vi "MS-2000 Stage Engine.vi"(0 "MS-2000 Notifier Name":string="MS2000", 11 "COM Port":string[](array[string])) -> ()   [LabVIEW 2020]
uses:
  Stages Controls/Stage Notifier Element.ctl
  Stages Controls/Stage Actions.ctl
  Stages Controls/Stage Status.ctl
  <vilib>/Instr/_visa.llb/VISA Configure Serial Port (Instr).vi
panel:
  out "Last Error":errorcluster
  in  "Get Position":bool
  in  "XY Step Size (µm)":dbl format="%#_4g"
  in  "Y Position (µm)":dbl format="%#_4g"
  in  "X Position (µm)":dbl format="%#_4g"
  in  "Home":bool
  in  "Right":bool
  in  "Left":bool
  in  "Down":bool
  in  "Halt":bool
  in  "Up":bool
  in  "Quit":bool
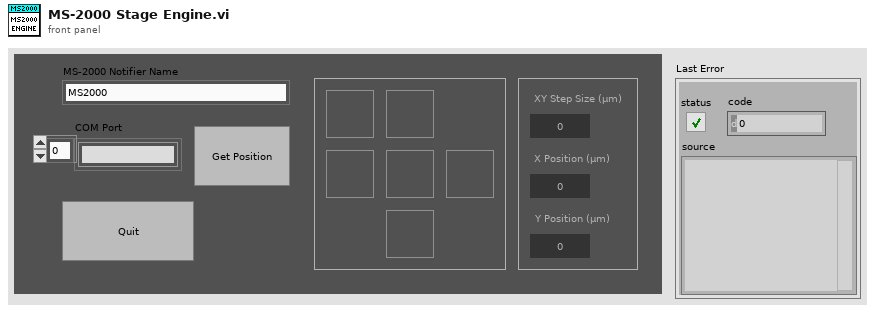
[diagram p1: front panel]
types:
  T1 = typedef "Stage Notifier Element.ctl" = cluster{"Action":T2, "Axis":bool[], "Setpoint":dbl[], "Velocity":dbl, "Cmd Recvd?":bool, "Position":dbl[], "Status":T3, "Misc":variant}
  T2 = typedef "Stage Actions.ctl" = enum16{"Get Position", "MVR", "MOVE", "HALT", "ONTARGET", "ERROR", "REFERENCE", "INIT", "VELOCITY", "STATUS", "EXIT", "HOME", "ZEROPOS", "NANOPOS", "ANALOG", "QUIT"}
  T3 = typedef "Stage Status.ctl" = enum16{"Error", "Abort", "Busy", "On Target"}
  T4 = enum32{"Invalid", "Standard", "Closed", "Hidden", "Minimized", "Maximized"}
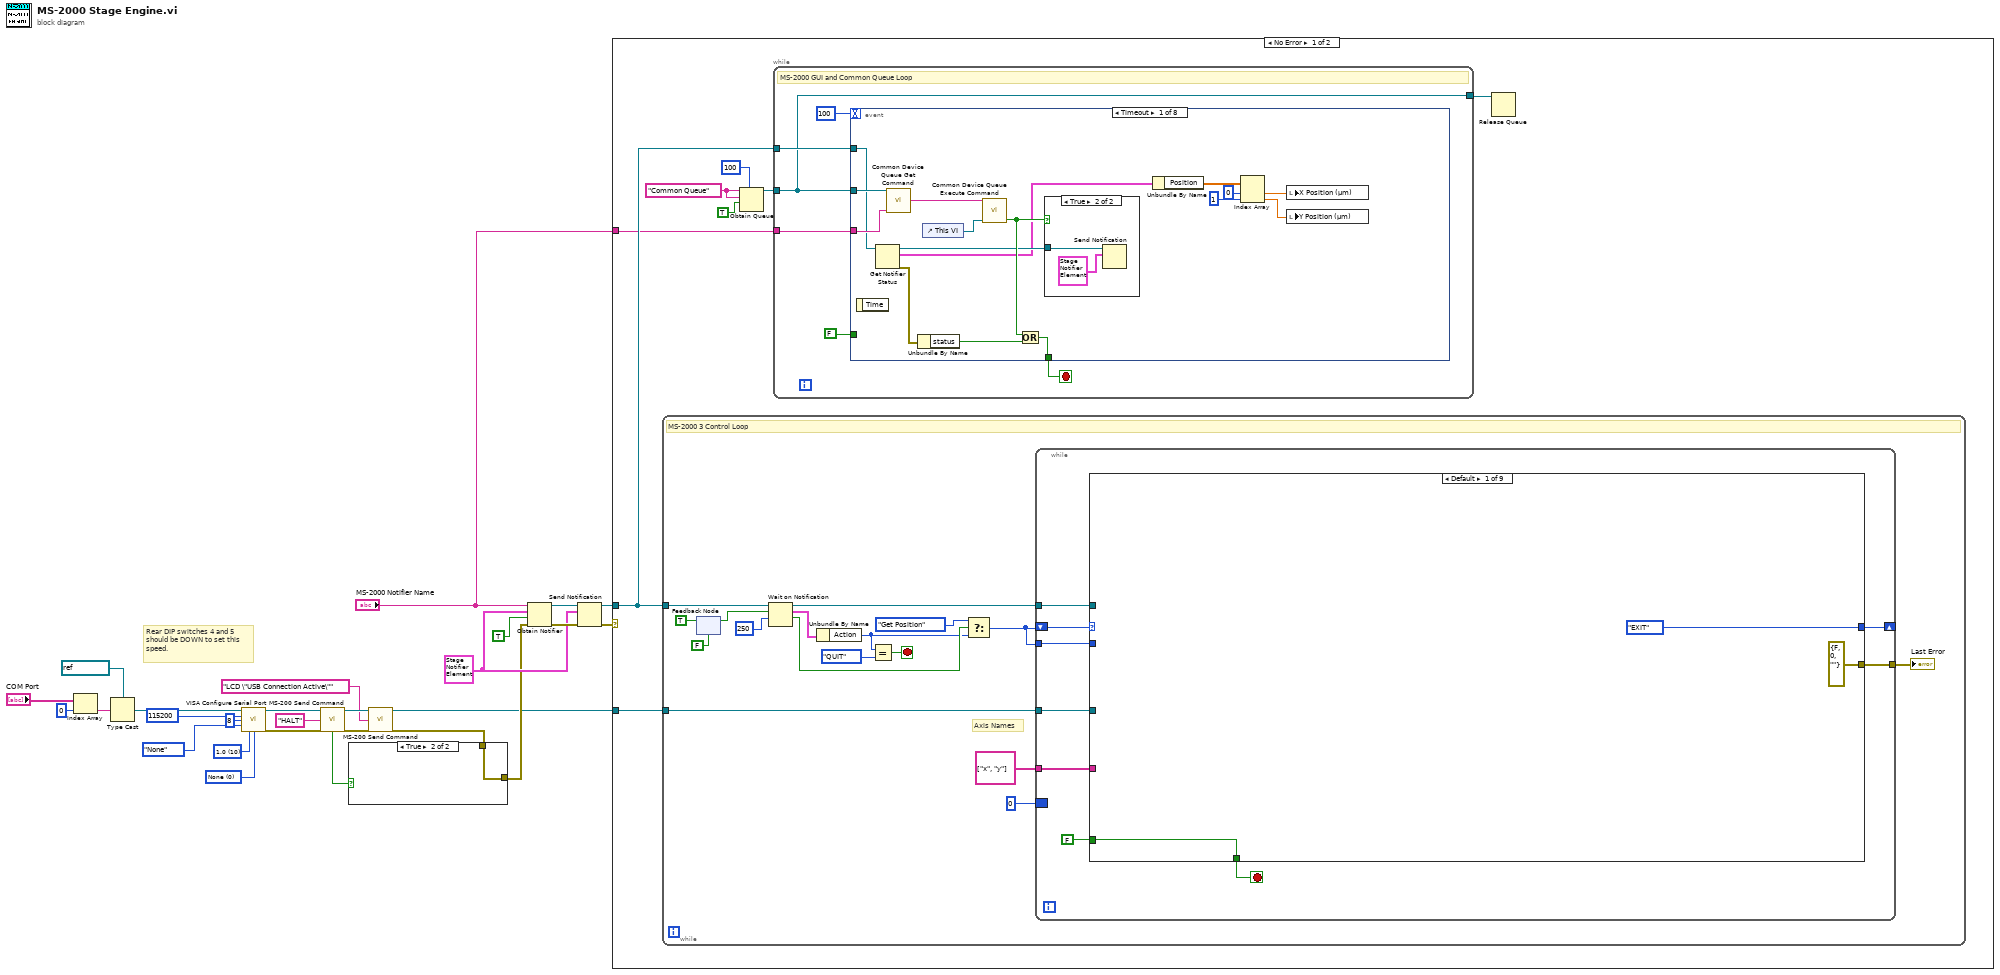
[diagram p0: block diagram]
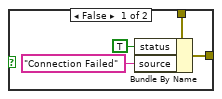
[diagram p2: hidden frame]
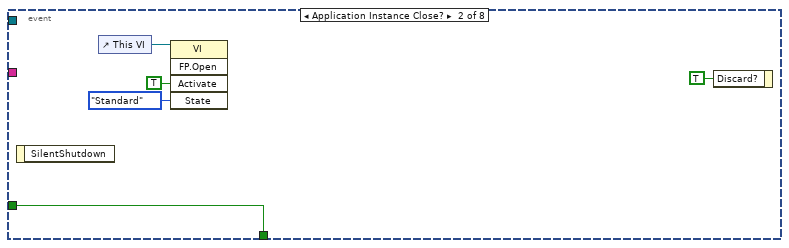
[diagram p4: hidden frame]
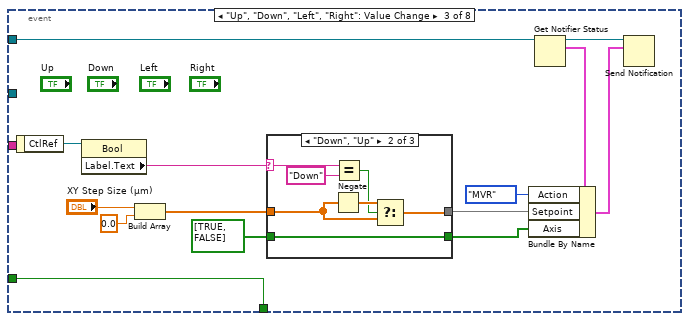
[diagram p5: hidden frame]
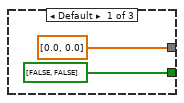
[diagram p6: hidden frame]
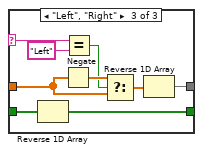
[diagram p7: hidden frame]
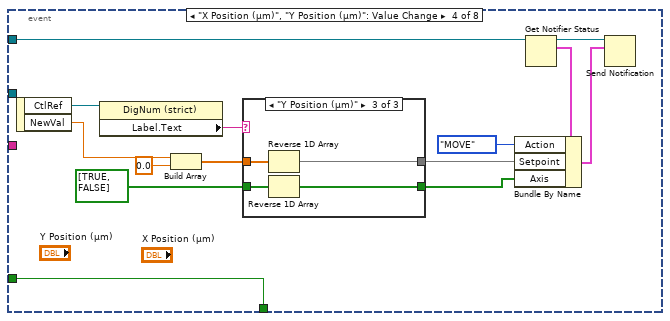
[diagram p8: hidden frame]
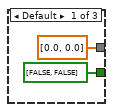
[diagram p9: hidden frame]
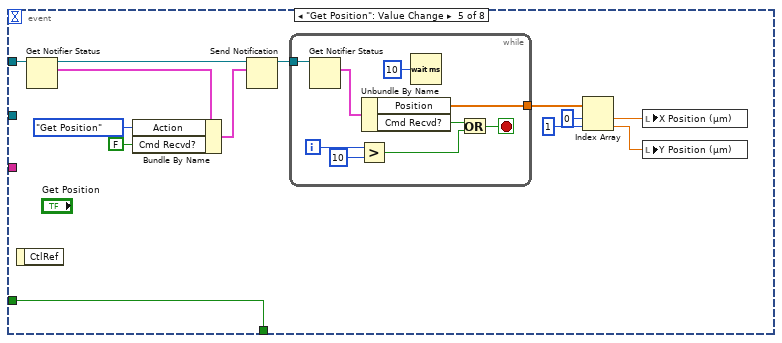
[diagram p11: hidden frame]
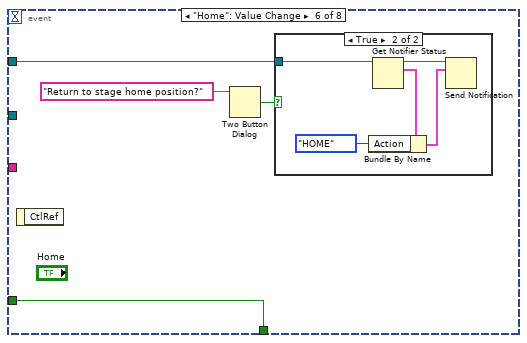
[diagram p12: hidden frame]
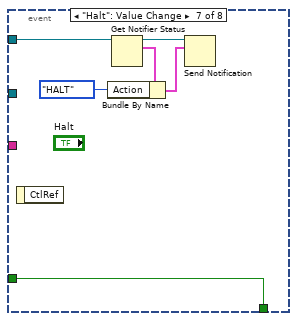
[diagram p14: hidden frame]
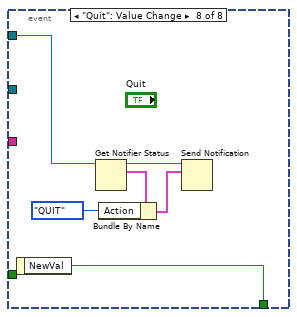
[diagram p15: hidden frame]
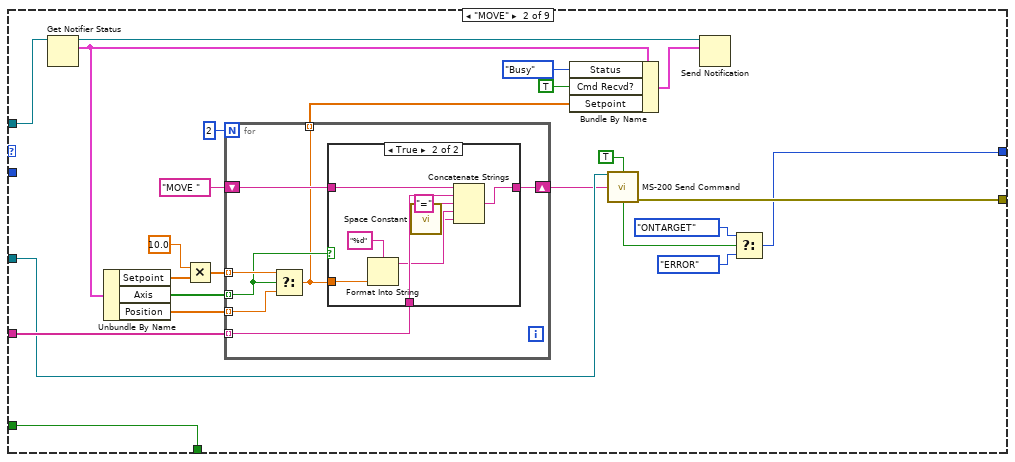
[diagram p16: hidden frame]
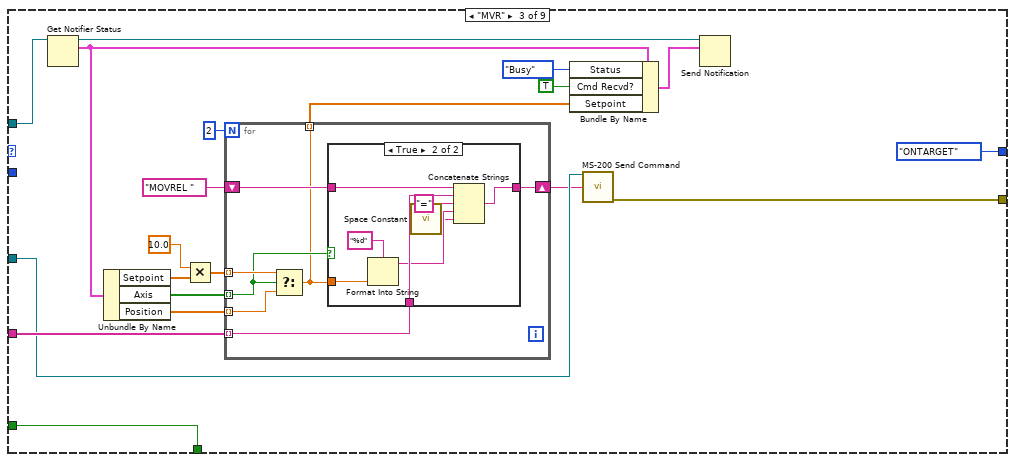
[diagram p18: hidden frame]
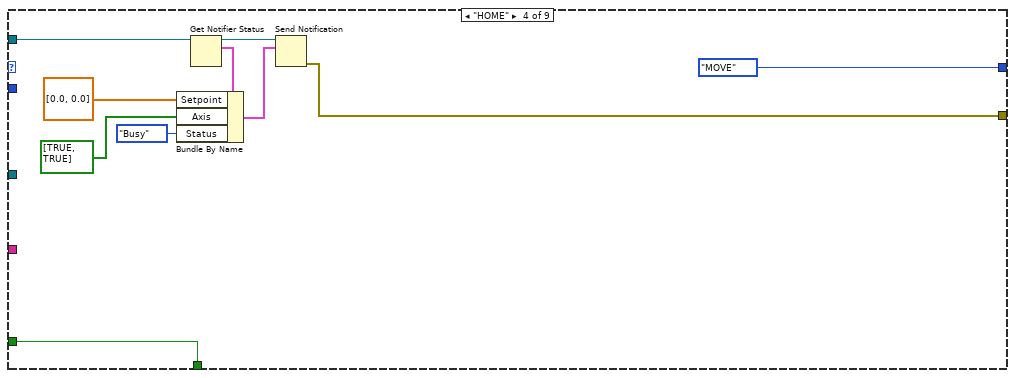
[diagram p20: hidden frame]
diagram:
  w18 = u16 0 items=["None", "XON/XOFF", "RTS/CTS", "XON/XOFF & RTS/CTS", "DTR/DSR", "XON/XOFF & DTR/DSR"] ("flow control (0:none)")
  w20 = u16 10 items=["1.0"=10, "1.5"=15, "2.0"=20] ("stop bits (10: 1 bit)")
  w22 = T1 {"Action"=enum."Get Position", "Axis"=[], "Setpoint"=[], "Velocity"=0.5, "Cmd Recvd?"=FALSE, "Position"=[], "Status"=enum."On Target", "Misc"=variant} ("Stage Status")
  # "Rear DIP switches 4 and 5 should be DOWN to set this speed."
  n1 = Index Array(array="COM Port", index=0) -> (element=w2:string)
  n2 = Type Cast(type=refnum<visa-resource-name> "COM5" ("VISA resource name"), x=w2) -> (*(type *) &x=w1:refnum<visa-resource-name>)
  n3 = call-poly "VISA Configure Serial Port"("VISA resource name"=w1, "baud rate (9600)"=u32 115200, "data bits (8)"=u16 8, "parity (0:none)"=enum16{"None", "Odd", "Even", "Mark", "Space"}."None", "stop bits (10: 1 bit)"=w20, "flow control (0:none)"=w18) -> ("VISA resource name out"=w15:refnum<visa-resource-name>, "error out"=w14:errorcluster)  [unwired: 8 in]
  n4 = call "MS-200 Send Command.vi"("VISA Ref"=w15, "Command"="HALT", "Error In"=w14) -> ("VISA Ref Dup"=w10:refnum<visa-resource-name>, "Cmd Success"=w12:bool, "Error Out"=w9:errorcluster)  [unwired: 9 in, 1 out]
  n5 = call "MS-200 Send Command.vi"("VISA Ref"=w10, "Command"="LCD \"USB Connection Active\"", "Error In"=w9) -> ("VISA Ref Dup"=w7:refnum<visa-resource-name>, "Error Out"=w6:errorcluster)  [unwired: 9 in, 2 out]
  n6 = case shown="True" w12 {
    tunnel: w6 -> [w31 w32]
    tunnel: [w28 w32] -> w11
    frame False {
      n7 = Bundle By Name(cluster=w31, "status"=TRUE, "source"="Connection Failed") -> (w28:errorcluster)
    }
    frame True {
    }
  }
  n8 = Obtain Notifier(name (unnamed)="MS-2000 Notifier Name", notification data type=w22, create if not found? (T)=TRUE, error in (no error)=w11) -> (notifier out=w26:refnum<notifier>, error out=w25:errorcluster)  [unwired: 1 out]
  n9 = Send Notification(notification=w22, notifier=w26, error in (no error)=w25) -> (notifier out=w23:refnum<notifier>, error out=w24:errorcluster)
  n10 = case shown="No Error" w24 {
    selector: w24 -> [_ w364]
    tunnel: w23 -> [w36 w365]
    tunnel: w7 -> [w40 w366]
    tunnel: "MS-2000 Notifier Name" -> [w35 _]
    frame No Error {
      w39 = "Common Queue" ("Unique Notifier Name")
      n11 = while {
        tunnel: w36 -> [w183]
        tunnel: w40 -> [w180]
        stop <- w179 stop-if-true
        # "Axis Names"
        # "MS-2000 3 Control Loop"
        n12 = feedback-in #1(TRUE ("ignore previous (F)")) -> ()
        n13 = feedback #1(FALSE ("ignore previous (F)")) -> (w174:bool)
        n14 = Wait on Notification(notifier=w183, ignore previous (F)=w174, timeout in ms (-1)=250) -> (notifier out=w182:refnum<notifier>, notification=w178:T1, timed out?=w172:bool)  [unwired: 1 in, 1 out]
        n15 = Unbundle By Name(w178) -> ("Action"=w170:T2)
        n16 = Equal?(x=w170, y=Stage_Actions."QUIT") -> (x = y?=w179:bool)
        n17 = Select(t=Stage_Actions."Get Position", s=w172, f=w170) -> (s? t:f=w169:T2)
        n18 = while {
          tunnel: w182 -> [w192]
          tunnel: w180 -> [w190]
          shift-right: [w189] -> _
          shift-left: w169 -> [w191]
          tunnel: w169 -> [w186]
          border: 0 -> [_]
          tunnel: string[] ["x", "y"] -> [w185]
          tunnel: [w184] -> w167
          stop <- w187 stop-if-true
          n19 = case shown="Default" w191 {
            selector: w191 -> [_ _ _ _ _ _ _ w344 _]
            tunnel: w192 -> [_ w215 w251 w277 w289 w314 w337 w346 w357]
            tunnel: w190 -> [_ w204 w239 _ w288 w309 w329 _ w355]
            tunnel: [Stage_Actions."EXIT" ("y") w196 Stage_Actions."ONTARGET" ("y") Stage_Actions."MOVE" ("y") w291 w311 w334 Stage_Actions."EXIT" ("y") Stage_Actions."QUIT" ("y")] -> w189
            tunnel: FALSE -> [w195 w219 w255 w275 _ w315 w331 _ _]
            tunnel: [w195 w219 w255 w275 w283 w315 w331 TRUE TRUE] -> w187
            tunnel: w186 -> [_ _ _ _ _ w310 _ _ _]
            tunnel: w185 -> [_ w206 w241 _ _ _ _ _ _]
            tunnel: [errorcluster {"status"=FALSE, "code"=0, "source"=""} ("error out") w202 w237 w272 w282 w304 w326 errorcluster {"status"=FALSE, "code"=0, "source"=""} ("Error Out") w352] -> w184
            frame Default {
            }
            frame "MOVE" {
              n20 = Get Notifier Status(notifier=w215) -> (notifier out=w217:refnum<notifier>, current notification=w212:T1)  [unwired: 1 in, 3 out]
              n21 = Unbundle By Name(w212) -> ("Setpoint"=w210:dbl[], "Axis"=w213:bool[], "Position"=w205:dbl[])
              n22 = Multiply(x=10.0, y=w210) -> (x*y=w208:dbl[])
              n23 = for {
                N: 2 -> [_]
                tunnel: w213 -> [w224] mode=indexing
                tunnel: w205 -> [w225] mode=indexing
                tunnel: w208 -> [w226] mode=indexing
                shift-right: [w222] -> w203
                shift-left: "MOVE " -> [w223]
                tunnel: [w220] -> w211 mode=indexing
                tunnel: w206 -> [w221] mode=indexing
                n24 = Select(t=w226, s=w224, f=w225) -> (s? t:f=w220:dbl)
                n25 = case shown="True" w224 {
                  tunnel: w223 -> [w227 w233]
                  tunnel: [w227 w228] -> w222
                  tunnel: w221 -> [_ w232]
                  tunnel: w220 -> [_ w235]
                  frame False {
                  }
                  frame True {
                    n26 = Format Into String(format string="%d", w235) -> (resulting string=w230:string)  [unwired: 2 in, 1 out]
                    n27 = call <vilib>:"Space Constant.vi"() -> ("String"=w229:string)
                    n28 = Concatenate Strings(w233, w232, "=" ("string"), w230, w229) -> (w228:string)
                  }
                }
              }
              n29 = Bundle By Name(cluster=w212, "Status"=Stage_Status."Busy", "Cmd Recvd?"=TRUE, "Setpoint"=w211) -> (w216:T1)
              n30 = call "MS-200 Send Command.vi"("VISA Ref"=w204, "Wait for Reply (T)"=TRUE, "Command"=w203) -> ("Cmd Success"=w199:bool, "Error Out"=w202:errorcluster)  [unwired: 9 in, 2 out]
              n31 = Send Notification(notification=w216, notifier=w217) -> ()  [unwired: 1 in, 2 out]
              n32 = Select(t=Stage_Actions."ONTARGET" ("y"), s=w199, f=Stage_Actions."ERROR") -> (s? t:f=w196:T2)
            }
            frame "MVR" {
              n33 = Get Notifier Status(notifier=w251) -> (notifier out=w253:refnum<notifier>, current notification=w247:T1)  [unwired: 1 in, 3 out]
              n34 = Unbundle By Name(w247) -> ("Setpoint"=w245:dbl[], "Axis"=w248:bool[], "Position"=w240:dbl[])
              n35 = Multiply(x=10.0, y=w245) -> (x*y=w243:dbl[])
              n36 = for {
                N: 2 -> [_]
                tunnel: w248 -> [w260] mode=indexing
                tunnel: w240 -> [w261] mode=indexing
                tunnel: w243 -> [w262] mode=indexing
                shift-right: [w258] -> w238
                shift-left: "MOVREL " -> [w259]
                tunnel: [w256] -> w246 mode=indexing
                tunnel: w241 -> [w257] mode=indexing
                n37 = Select(t=w262, s=w260, f=w261) -> (s? t:f=w256:dbl)
                n38 = case shown="True" w260 {
                  tunnel: w259 -> [w263 w269]
                  tunnel: [w263 w264] -> w258
                  tunnel: w257 -> [_ w268]
                  tunnel: w256 -> [_ w271]
                  frame False {
                  }
                  frame True {
                    n39 = Format Into String(format string="%d", w271) -> (resulting string=w266:string)  [unwired: 2 in, 1 out]
                    n40 = call <vilib>:"Space Constant.vi"() -> ("String"=w265:string)
                    n41 = Concatenate Strings(w269, w268, "=" ("string"), w266, w265) -> (w264:string)
                  }
                }
              }
              n42 = Bundle By Name(cluster=w247, "Status"=Stage_Status."Busy", "Cmd Recvd?"=TRUE, "Setpoint"=w246) -> (w252:T1)
              n43 = call "MS-200 Send Command.vi"("VISA Ref"=w239, "Command"=w238) -> ("Error Out"=w237:errorcluster)  [unwired: 10 in, 3 out]
              n44 = Send Notification(notification=w252, notifier=w253) -> ()  [unwired: 1 in, 2 out]
            }
            frame "HOME" {
              n45 = Get Notifier Status(notifier=w277) -> (notifier out=w279:refnum<notifier>, current notification=w280:T1)  [unwired: 1 in, 3 out]
              n46 = Bundle By Name(cluster=w280, "Setpoint"=dbl[] [0.0, 0.0], "Axis"=bool[] [TRUE, TRUE], "Status"=Stage_Status."Busy") -> (w278:T1)
              n47 = Send Notification(notification=w278, notifier=w279) -> (error out=w272:errorcluster)  [unwired: 1 in, 1 out]
            }
            frame "ONTARGET" {
              n48 = feedback #2() -> (w296:i32)
              n49 = call "MS-200 Send Command.vi"("VISA Ref"=w288, "Command"="/") -> ("Reply"=w286:string, "Error Out"=w282:errorcluster)  [unwired: 10 in, 2 out]
              n50 = Increment(x=w296) -> (x+1=w295:i32)
              n51 = feedback-in #2(w295) -> ()
              n52 = Equal?(x="N", y=w286) -> (x = y?=w284:bool)
              n53 = Less Or Equal?(x=w295, y=250) -> (x <= y?=w283:bool)
              n54 = Select(t=Stage_Actions."EXIT" ("y"), s=w284, f=Stage_Actions."Get Position" ("y")) -> (s? t:f=w293:T2)
              n55 = Select(t=Stage_Status."On Target" ("Status"), s=w284, f=Stage_Status."Busy" ("Status")) -> (s? t:f=w297:T3)
              n56 = Get Notifier Status(notifier=w289) -> (notifier out=w301:refnum<notifier>, current notification=w302:T1)  [unwired: 1 in, 3 out]
              n57 = Bundle By Name(cluster=w302, "Status"=w297) -> (w300:T1)
              n58 = Send Notification(notification=w300, notifier=w301) -> ()  [unwired: 1 in, 2 out]
              n59 = Select(t=w293, s=w283, f=Stage_Actions."ERROR") -> (s? t:f=w291:T2)
            }
            frame "Get Position" {
              n60 = call "MS-200 Send Command.vi"("VISA Ref"=w309, "Command"="WHERE X Y") -> ("Reply"=w306:string, "Error Out"=w307:errorcluster)  [unwired: 10 in, 2 out]
              n61 = call "MS-2000 Read Positions.vi"("WHERE Reply"=w306, "Error In"=w307) -> ("Positions um"=w305:dbl[], "Error Out"=w304:errorcluster)  [unwired: 11 in, 1 out]
              n62 = Get Notifier Status(notifier=w314) -> (notifier out=w316:refnum<notifier>, current notification=w313:T1)  [unwired: 1 in, 3 out]
              n63 = case shown="Default" w310 {
                tunnel: w313 -> [w320 w325]
                tunnel: [w319 w324] -> w312
                tunnel: w305 -> [w318 w323]
                tunnel: [Stage_Actions."ONTARGET" ("y") Stage_Actions."EXIT" ("y")] -> w311
                frame Default {
                  n64 = Bundle By Name(cluster=w320, "Position"=w318) -> (w319:T1)
                }
                frame "Get Position", "HALT" {
                  n65 = Bundle By Name(cluster=w325, "Position"=w323, "Cmd Recvd?"=TRUE) -> (w324:T1)
                }
              }
              n66 = Send Notification(notification=w312, notifier=w316) -> ()  [unwired: 1 in, 2 out]
            }
            frame "HALT" {
              n67 = call "MS-200 Send Command.vi"("VISA Ref"=w329, "Command"="HALT") -> ("Cmd Success"=w327:bool, "Error Out"=w326:errorcluster)  [unwired: 10 in, 2 out]
              n68 = Select(t=Stage_Status."Abort" ("Status"), s=w327, f=Stage_Status."Error" ("Status")) -> (s? t:f=w330:T3)
              n69 = Select(t=Stage_Actions."Get Position" ("y"), s=w327, f=Stage_Actions."ERROR" ("y")) -> (s? t:f=w334:T2)
              n70 = Get Notifier Status(notifier=w337) -> (notifier out=w340:refnum<notifier>, current notification=w341:T1)  [unwired: 1 in, 3 out]
              n71 = Bundle By Name(cluster=w341, "Status"=w330, "Cmd Recvd?"=TRUE) -> (w339:T1)
              n72 = Send Notification(notification=w339, notifier=w340) -> ()  [unwired: 1 in, 2 out]
            }
            frame "ERROR".."EXIT" {
              n73 = case shown="\"ERROR\"" w344 {
                tunnel: w346 -> [_ w351]
                frame Default {
                }
                frame "ERROR" {
                  n74 = Get Notifier Status(notifier=w351) -> (notifier out=w348:refnum<notifier>, current notification=w350:T1)  [unwired: 1 in, 3 out]
                  n75 = Bundle By Name(cluster=w350, "Status"=Stage_Status."Error") -> (w347:T1)
                  n76 = Send Notification(notification=w347, notifier=w348) -> ()  [unwired: 1 in, 2 out]
                }
              }
            }
            frame "QUIT" {
              n77 = Release Notifier(notifier=w357, force destroy? (F)=TRUE) -> ()  [unwired: 1 in, 3 out]
              n78 = VISA Close(VISA resource name=w355) -> (error out=w352:errorcluster)  [unwired: 1 in]
            }
          }
        }
        "Last Error" <- w167
      }
      n79 = Obtain Queue(max queue size (-1, unlimited)=100, name (unnamed)=w39, element data type=w39, create if not found? (T)=TRUE) -> (queue out=w37:refnum<queue>)  [unwired: 1 in, 2 out]
      n80 = while {
        tunnel: w37 -> [w41]
        tunnel: w35 -> [w44]
        tunnel: w36 -> [w45]
        tunnel: [w41] -> w33
        stop <- w43 stop-if-true
        # "MS-2000 GUI and Common Queue Loop"
        n81 = event shown="[0] Timeout" {
          selector: _ -> [_ _ _ _ _ _ _ _]
          dyn-events: _ -> [_ _ _ _ _ _ _ _]
          timeout: 100 -> [_ _ _ _ _ _ _ _]
          tunnel: w41 -> [w56 _ _ _ _ _ _ _]
          tunnel: w45 -> [w53 _ w76 w108 w135 w146 w159 w166]
          tunnel: w44 -> [w55 _ _ _ _ _ _ _]
          tunnel: [w54 w69 w79 w115 w136 w148 w160 w162] -> w43
          tunnel: FALSE -> [_ w69 w79 w115 w136 w148 w160 _]
          event Timeout {
            n82 = event-data() -> ()  [unwired: 1 in, 1 out]
            n83 = Get Notifier Status(notifier=w53) -> (notifier out=w57:refnum<notifier>, current notification=w47:T1, error out=w62:errorcluster)  [unwired: 1 in, 2 out]
            n84 = call "Common Device Queue Get Command.vi"("Common Queue"=w56, "Notifier Name"=w55) -> ("Command"=w61:string)  [unwired: 12 in, 1 out]
            n85 = Unbundle By Name(w62) -> ("status"=w59:bool)
            n86 = control-ref of="This VI"() -> (w60:refnum<vi>)
            n87 = call "Common Device Queue Execute Command.vi"("Common Command"=w61, "VI Refnum"=w60) -> ("Quit?"=w58:bool)  [unwired: 12 in, 1 out]
            n88 = Or(x=w58, y=w59) -> (x .or. y?=w54:bool)
            n89 = case shown="True" w58 {
              tunnel: w57 -> [_ w64]
              frame False {
              }
              frame True {
                n90 = Send Notification(notification=T1 {"Action"=enum."QUIT", "Axis"=[], "Setpoint"=[], "Velocity"=0.5, "Cmd Recvd?"=FALSE, "Position"=[], "Status"=enum."Error", "Misc"=variant} ("Stage Status"), notifier=w64) -> ()  [unwired: 1 in, 2 out]
              }
            }
            n91 = Unbundle By Name(w47) -> ("Position"=w48:dbl[])
            n92 = Index Array(array=w48, index #1=0 ("index"), index #2=1 ("index")) -> (element #1=w52:dbl, element #2=w51:dbl)
            n93 = local write "X Position (µm)"(w52) -> ()
            n94 = local write "Y Position (µm)"(w51) -> ()
          }
          event Application Instance Close? {
            n95 = event-data() -> ()  [unwired: 1 in, 1 out]
            n96 = control-ref of="This VI"() -> (w66:refnum<vi>)
            n97 = invoke class="VI" method="FP.Open"(reference=w66, "Activate"=TRUE ("Activate?"), "State"=T4."Standard") -> ()  [unwired: 2 in, 5 out]
            n98 = event-data("Discard?"=TRUE) -> ()  [unwired: 1 in, 1 out]
          }
          event "Up", "Down", "Left", "Right": Value Change {
            n99 = event-data() -> ("CtlRef"=w78:refnum<vi>)  [unwired: 1 in]
            n100 = property class="Bool"(reference=w78) -> ("Label.Text"=w83:string)  [unwired: 1 in, 2 out]
            n101 = Build Array("XY Step Size (µm)", 0.0 ("element")) -> (w81:dbl[])
            n102 = case shown="\"Down\", \"Up\"" w83 {
              selector: w83 -> [_ w92 w98]
              tunnel: w81 -> [_ w89 w97]
              tunnel: bool[] [TRUE, FALSE] -> [_ w86 w95]
              tunnel: [dbl[] [0.0, 0.0] w88 w94] -> w74
              tunnel: [bool[] [FALSE, FALSE] w86 w93] -> w73
              frame Default {
              }
              frame "Down", "Up" {
                n103 = Negate(x=w89) -> (-x=w90:dbl[])
                n104 = Equal?(x=w92, y="Down") -> (x = y?=w87:bool)
                n105 = Select(t=w90, s=w87, f=w89) -> (s? t:f=w88:dbl[])
              }
              frame "Left", "Right" {
                n106 = Reverse 1D Array(array=w95) -> (reversed array=w93:bool[])
                n107 = Negate(x=w97) -> (-x=w100:dbl[])
                n108 = Equal?(x=w98, y="Left") -> (x = y?=w99:bool)
                n109 = Select(t=w100, s=w99, f=w97) -> (s? t:f=w96:dbl[])
                n110 = Reverse 1D Array(array=w96) -> (reversed array=w94:dbl[])
              }
            }
            n111 = Get Notifier Status(notifier=w76) -> (notifier out=w71:refnum<notifier>, current notification=w75:T1)  [unwired: 1 in, 3 out]
            n112 = Bundle By Name(cluster=w75, "Action"=Stage_Actions."MVR", "Setpoint"=w74, "Axis"=w73) -> (w70:T1)
            n113 = Send Notification(notification=w70, notifier=w71) -> ()  [unwired: 1 in, 2 out]
          }
          event "X Position (µm)", "Y Position (µm)": Value Change {
            n114 = event-data() -> ("CtlRef"=w110:refnum<vi>, "NewVal"=w109:dbl)  [unwired: 1 in]
            n115 = property class="DigNum (strict)"(reference=w110) -> ("Label.Text"=w113:string)  [unwired: 1 in, 2 out]
            n116 = Build Array(w109, 0.0 ("element")) -> (w114:dbl[])
            n117 = case shown="\"Y Position (µm)\"" w113 {
              tunnel: w114 -> [_ w119 w123]
              tunnel: bool[] [TRUE, FALSE] -> [_ w118 w122]
              tunnel: [dbl[] [0.0, 0.0] w119 w121] -> w105
              tunnel: [bool[] [FALSE, FALSE] w118 w120] -> w104
              frame Default {
              }
              frame "X Position (µm)" {
              }
              frame "Y Position (µm)" {
                n118 = Reverse 1D Array(array=w123) -> (reversed array=w121:dbl[])
                n119 = Reverse 1D Array(array=w122) -> (reversed array=w120:bool[])
              }
            }
            n120 = Get Notifier Status(notifier=w108) -> (notifier out=w107:refnum<notifier>, current notification=w106:T1)  [unwired: 1 in, 3 out]
            n121 = Bundle By Name(cluster=w106, "Action"=Stage_Actions."MOVE", "Setpoint"=w105, "Axis"=w104) -> (w102:T1)
            n122 = Send Notification(notification=w102, notifier=w107) -> ()  [unwired: 1 in, 2 out]
          }
          event "Get Position": Value Change {
            n123 = event-data() -> ()  [unwired: 1 in, 1 out]
            n124 = Get Notifier Status(notifier=w135) -> (notifier out=w134:refnum<notifier>, current notification=w133:T1)  [unwired: 1 in, 3 out]
            n125 = Bundle By Name(cluster=w133, "Action"=Stage_Actions."Get Position", "Cmd Recvd?"=FALSE) -> (w130:T1)
            n126 = Send Notification(notification=w130, notifier=w134) -> (notifier out=w129:refnum<notifier>)  [unwired: 1 in, 1 out]
            n127 = while {
              tunnel: w129 -> [w145]
              tunnel: [w137] -> w128
              i -> [w141]
              stop <- w138 stop-if-true
              n128 = Get Notifier Status(notifier=w145) -> (current notification=w144:T1)  [unwired: 1 in, 4 out]
              n129 = Greater?(x=w141, y=10) -> (0:w139:bool)
              n130 = Unbundle By Name(w144) -> ("Position"=w137:dbl[], "Cmd Recvd?"=w140:bool)
              n131 = Wait (ms)(milliseconds to wait=u32 10) -> ()  [unwired: 1 out]
              n132 = Or(x=w140, y=w139) -> (x .or. y?=w138:bool)
            }
            n133 = Index Array(array=w128, index #1=0 ("index"), index #2=1 ("index")) -> (element #1=w125:dbl, element #2=w124:dbl)
            n134 = local write "X Position (µm)"(w125) -> ()
            n135 = local write "Y Position (µm)"(w124) -> ()
          }
          event "Home": Value Change {
            n136 = event-data() -> ()  [unwired: 1 in, 1 out]
            n137 = Two Button Dialog(message="Return to stage home position?") -> (T button?=w147:bool)  [unwired: 2 in]
            n138 = case shown="True" w147 {
              tunnel: w146 -> [_ w154]
              frame False {
              }
              frame True {
                n139 = Get Notifier Status(notifier=w154) -> (notifier out=w153:refnum<notifier>, current notification=w152:T1)  [unwired: 1 in, 3 out]
                n140 = Bundle By Name(cluster=w152, "Action"=Stage_Actions."HOME") -> (w151:T1)
                n141 = Send Notification(notification=w151, notifier=w153) -> ()  [unwired: 1 in, 2 out]
              }
            }
          }
          event "Halt": Value Change {
            n142 = event-data() -> ()  [unwired: 1 in, 1 out]
            n143 = Get Notifier Status(notifier=w159) -> (notifier out=w158:refnum<notifier>, current notification=w157:T1)  [unwired: 1 in, 3 out]
            n144 = Bundle By Name(cluster=w157, "Action"=Stage_Actions."HALT") -> (w156:T1)
            n145 = Send Notification(notification=w156, notifier=w158) -> ()  [unwired: 1 in, 2 out]
          }
          event "Quit": Value Change {
            n146 = event-data() -> ("NewVal"=w162:bool)  [unwired: 1 in]
            n147 = Get Notifier Status(notifier=w166) -> (notifier out=w165:refnum<notifier>, current notification=w164:T1)  [unwired: 1 in, 3 out]
            n148 = Bundle By Name(cluster=w164, "Action"=Stage_Actions."QUIT") -> (w163:T1)
            n149 = Send Notification(notification=w163, notifier=w165) -> ()  [unwired: 1 in, 2 out]
          }
        }
      }
      n150 = Release Queue(queue=w33) -> ()  [unwired: 2 in, 3 out]
    }
    frame Error {
      n151 = VISA Close(VISA resource name=w366) -> ()  [unwired: 1 in, 1 out]
      n152 = Release Notifier(notifier=w365, force destroy? (F)=TRUE, error in (no error)=w364) -> (error out=w362:errorcluster)  [unwired: 2 out]
      n153 = Unbundle By Name(w362) -> ("source"=w359:string)
      n154 = Concatenate Strings("Pro Scan 3 Error", "\r", w359) -> (w358:string)
      n155 = One Button Dialog(message=w358) -> ()  [unwired: 1 in, 1 out]
    }
  }
